vi "Backup Notebook Content.vi"(8 "error in":errorcluster, 9 "Notebook Backup Path":path, 11 "Rich Text Box .NET Refnum":refnum<k24>) -> (0 "error out":errorcluster, 1 "Message":string)   [LabVIEW 2021, in "Notebook.lvlib"]
uses:
  Notebook.lvlib
  System.Windows.Forms
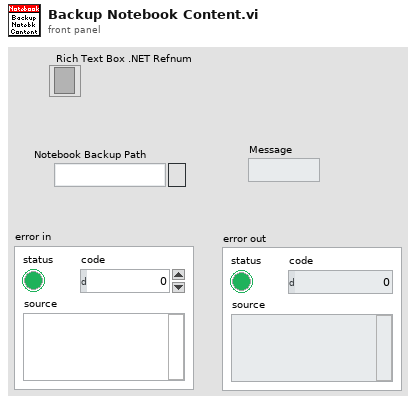
[diagram p1: front panel]
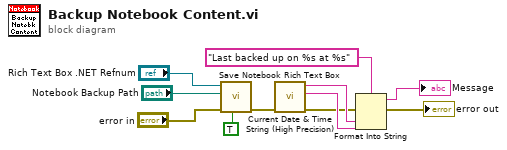
[diagram p0: block diagram]
diagram:
  n1 = call "Save Notebook Rich Text Box.vi"("Backup?"=TRUE, "Error In"="error in", "File Path Control"="Notebook Backup Path", ".NET Refnum in"="Rich Text Box .NET Refnum") -> ("Error Out"=w6:errorcluster)  [unwired: 4 in, 3 out]
  n2 = call "Current Date & Time String (High Precision).vi"("Error In"=w6) -> ("Error Out"=w7:errorcluster, "time string"=w9:string, "date string"=w8:string)  [unwired: 7 in, 1 out]
  n3 = Format Into String(format string="Last backed up on %s at %s", error in=w7, w8, w9) -> (resulting string=→"Message":string, error out=→"error out":errorcluster)  [unwired: 1 in]
